vi "get_output_retransmission_output_value.vi"(8 "error in (no error)":errorcluster, 11 "connection ID":refnum<k5>) -> (0 "error out":errorcluster, 2 "Value":dbl, 3 "connection ID out":refnum<k5>)   [LabVIEW 2018]
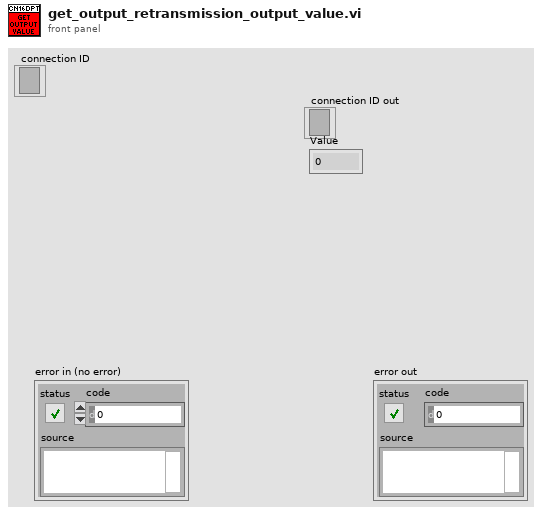
[diagram p1: front panel]
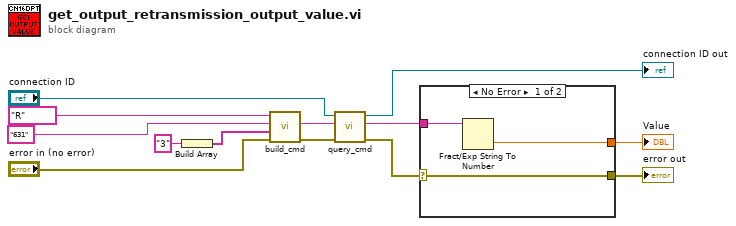
[diagram p0: block diagram]
diagram:
  n1 = Build Array("3") -> (w2:string[])
  n2 = call "build_cmd.vi"("error in (no error)"="error in (no error)", "Parameter list"=w2, "Command ID"="631", "Command class"="R") -> ("error out"=w10:errorcluster, "Command"=w9:string)  [unwired: 6 in]
  n3 = call "query_cmd.vi"("error in (no error)"=w10, "Command"=w9, "connection ID"="connection ID") -> ("error out"=w8:errorcluster, "Response"=w7:string, "connection ID out"=→"connection ID out":refnum<k5>)  [unwired: 6 in]
  n4 = case shown="No Error" w8 {
    selector: w8 -> [w14 w17]
    tunnel: w7 -> [w16 _]
    tunnel: [w15 _] -> w1
    tunnel: [w14 w17] -> w6
    frame No Error {
      n5 = Fract/Exp String To Number(string=w16) -> (number=w15:dbl)  [unwired: 3 in, 1 out]
    }
    frame Error {
    }
  }
  "error out" <- w6
  "Value" <- w1
